vi "HEWH Add Output Range to Error Code.vi"(6 "Range?":bool, 7 "Units":string="F", 9 "Value Max":dbl, 10 "Value Min":dbl, 11 "Input String":string) -> (3 "Display Range":string)   [LabVIEW 2020]
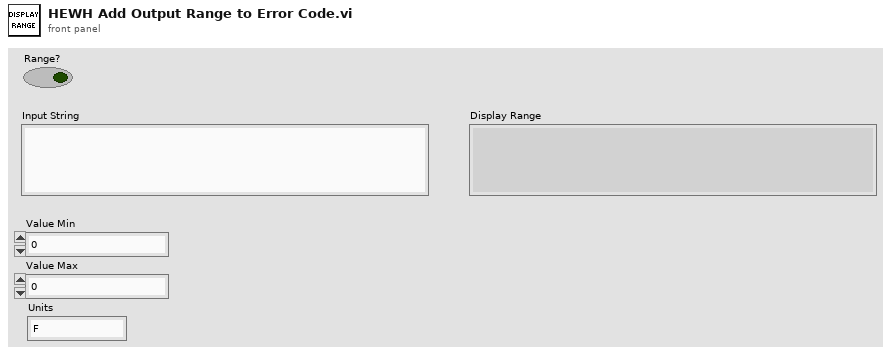
[diagram p1: front panel]
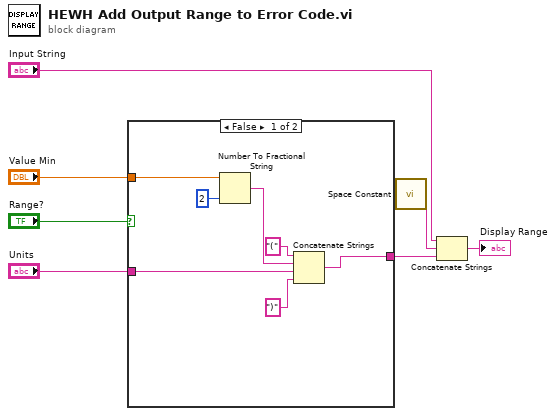
[diagram p0: block diagram]
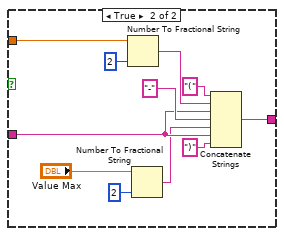
[diagram p2: hidden frame]
diagram:
  n1 = case shown="False" "Range?" {
    tunnel: "Units" -> [w10 w21]
    tunnel: "Value Min" -> [w8 w18]
    tunnel: [w9 w15] -> w2
    frame False {
      n2 = Number To Fractional String(number=w8, precision (6)=i16 2) -> (F-format string=w14:string)  [unwired: 2 in]
      n3 = Concatenate Strings("(", w14, w10, ")") -> (w9:string)
    }
    frame True {
      n4 = Number To Fractional String(number=w18, precision (6)=i16 2) -> (F-format string=w16:string)  [unwired: 2 in]
      n5 = Number To Fractional String(number="Value Max", precision (6)=i16 2) -> (F-format string=w17:string)  [unwired: 2 in]
      n6 = Concatenate Strings("(", w16, w21, "-", w17, w21, ")") -> (w15:string)
    }
  }
  n7 = call <vilib>:"Space Constant.vi"() -> ("String"=w3:string)
  n8 = Concatenate Strings("Input String", w3, w2) -> (→"Display Range":string)
